vi "LHF.DB.Mongo.Collection.Aggregate.vi"(6 "Extract _id (T)":bool=TRUE, 7 "return type":variant, 8 "error in (no error)":errorcluster, 9 "Operations":variant[](array[variant]), 10 "Collection":string, 11 "LHF.DB.Mongo in":refnum<class "LHF.DB.Mongo.lvclass">) -> (0 "error out":errorcluster, 1 "_id Array":string[](array[string]), 2 "Documents":variant[](array[variant]), 3 "LHF.DB.Mongo out":refnum<class "LHF.DB.Mongo.lvclass">)   [LabVIEW 2013, in "LHF.DB.Mongo.lvclass"]
doc: "return type: wire cluster of expected document output, then variant to data with documents output. use cluster element's name to choose what document field you're expecting\noperations: wire array of cluster variant, name the cluster variant with the desired aggregation operation as $project or $match then use element names to setup pipeline."
uses:
  LHF.DB.Mongo.lvclass
  C:/Users/Ricardo/Desktop/Projetos/LabVIEW-MongoDB/src/Driver/MongoDB.Bson.dll
  Driver/MongoDB.Bson.dll
  <userlib>/_OpenG.lib/string/string.llb/Trim Whitespace (String)__ogtk.vi
  <vilib>/Utility/VariantDataType/VariantType.lvlib
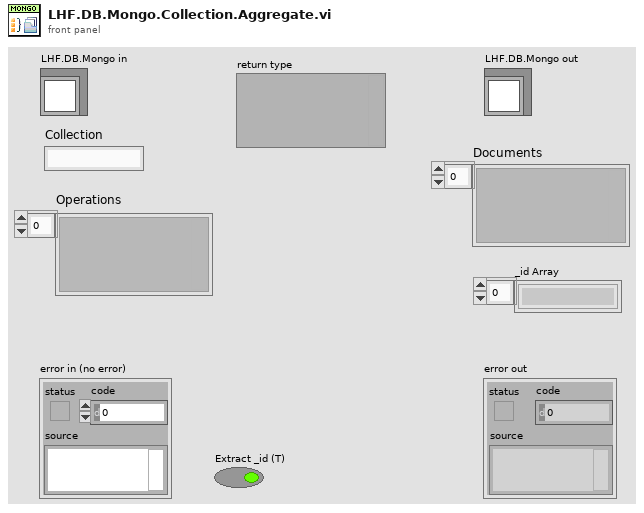
[diagram p1: front panel]
types:
  T1 = enum16{"$project", "$limit", "$skip", "$match", "$redact", "$unwind", "$group", "$sort", "$sample", "$geonear", "$lookup", "$out", "$indexstats"}
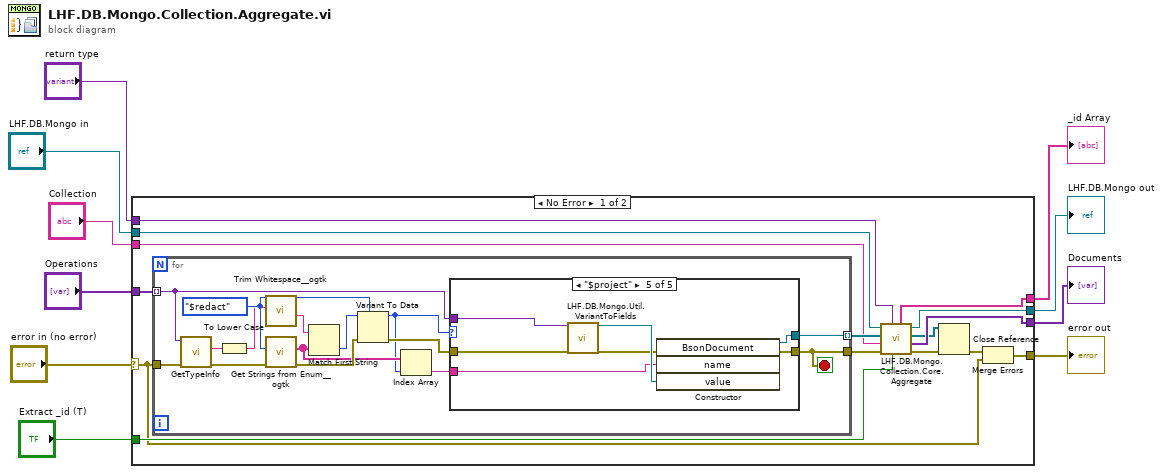
[diagram p0: block diagram]
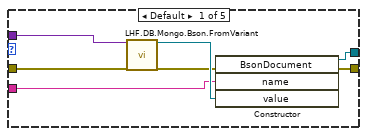
[diagram p2: hidden frame]
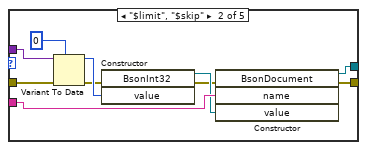
[diagram p3: hidden frame]
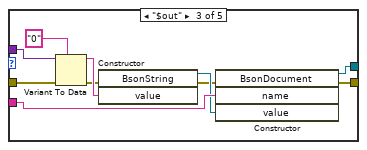
[diagram p4: hidden frame]
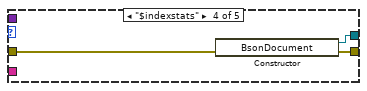
[diagram p5: hidden frame]
diagram:
  n1 = case shown="No Error" "error in (no error)" {
    selector: "error in (no error)" -> [w12 w79]
    tunnel: [w20 w79] -> w9
    tunnel: [w23 w78] -> w7
    tunnel: "LHF.DB.Mongo in" -> [w24 w78]
    tunnel: "Collection" -> [w19 _]
    tunnel: "Operations" -> [w25 _]
    tunnel: [w18 _] -> w4
    tunnel: "Extract _id (T)" -> [w17 _]
    tunnel: [w16 _] -> w2
    tunnel: "return type" -> [w11 _]
    frame No Error {
      n2 = for {
        tunnel: w25 -> [w38] mode=indexing
        tunnel: [w40] -> w21 mode=indexing
        tunnel: [w39] -> w22
        tunnel: w12 -> [w31]
        stop <- w39 stop-if-true
        w37 = T1."$redact"
        n3 = call <vilib>:"GetTypeInfo.vi"("error in (no error)"=w31, "Variant"=w38) -> ("error out"=w32:errorcluster, "Name"=w34:string)  [unwired: 5 in, 3 out]
        n4 = To Lower Case(string=w34) -> (all lower case string=w26:string)
        n5 = call-poly <userlib>:"Trim Whitespace__ogtk.vi"("String in"=w26) -> ("String out"=w35:string)  [unwired: 6 in]
        n6 = call <userlib>:"Get Strings from Enum__ogtk.vi"("error in (no error)"=w32, "Enum"=w37) -> ("error out"=w33:errorcluster, "Enum Strings"=w29:string[])  [unwired: 6 in, 2 out]
        n7 = Match First String(2:w29, 3:w35) -> (0:w36:i32)  [unwired: 1 out]
        n8 = Variant To Data(error in=w33, type=w37, Variant=w36) -> (data=w28:T1, error out=w30:errorcluster)
        n9 = Index Array(array=w29, index=w28) -> (element=w27:string)
        n10 = case shown="\"$project\"" w28 {
          tunnel: [w43 w53 w63 w70 w73] -> w40
          tunnel: [w42 w48 w58 w69 w72] -> w39
          tunnel: w30 -> [w46 w55 w65 w68 w77]
          tunnel: w38 -> [w47 w57 w67 _ w76]
          tunnel: w27 -> [w41 w54 w64 _ w71]
          frame Default {
            n11 = call "LHF.DB.Mongo.Bson.FromVariant.vi"("Variant"=w47, "error IO"=w46) -> ("BsonValue"=w45:refnum<k24>, "error IO 2"=w44:errorcluster)  [unwired: 16 in]
            n12 = constructor class="BsonDocument"(error in=w44, "name"=w41, "value"=w45) -> (reference out=w43:refnum<k24>, error out=w42:errorcluster)  [unwired: 2 in, 3 out]
          }
          frame "$limit", "$skip" {
            n13 = Variant To Data(error in=w55, type=0, Variant=w57) -> (data=w52:i32, error out=w51:errorcluster)
            n14 = constructor class="BsonInt32"(error in=w51, "value"=w52) -> (reference out=w50:refnum<k24>, error out=w49:errorcluster)  [unwired: 2 in, 2 out]
            n15 = constructor class="BsonDocument"(error in=w49, "name"=w54, "value"=w50) -> (reference out=w53:refnum<k24>, error out=w48:errorcluster)  [unwired: 2 in, 3 out]
          }
          frame "$out" {
            n16 = Variant To Data(error in=w65, type="0", Variant=w67) -> (data=w62:string, error out=w61:errorcluster)
            n17 = constructor class="BsonString"(error in=w61, "value"=w62) -> (reference out=w60:refnum<k24>, error out=w59:errorcluster)  [unwired: 2 in, 2 out]
            n18 = constructor class="BsonDocument"(error in=w59, "name"=w64, "value"=w60) -> (reference out=w63:refnum<k24>, error out=w58:errorcluster)  [unwired: 2 in, 3 out]
          }
          frame "$indexstats" {
            n19 = constructor class="BsonDocument"(error in=w68) -> (reference out=w70:refnum<k24>, error out=w69:errorcluster)  [unwired: 2 in, 1 out]
          }
          frame "$project" {
            n20 = call "LHF.DB.Mongo.Util.VariantToFields.vi"("projection type"=w76, "error in (no error)"=w77) -> ("BsonDocument"=w75:refnum<k24>, "error out"=w74:errorcluster)  [unwired: 16 in]
            n21 = constructor class="BsonDocument"(error in=w74, "name"=w71, "value"=w75) -> (reference out=w73:refnum<k24>, error out=w72:errorcluster)  [unwired: 2 in, 3 out]
          }
        }
      }
      n22 = call "LHF.DB.Mongo.Collection.Core.Aggregate.vi"("Extract _id"=w17, "type"=w11, "error in (no error)"=w22, "Collection"=w19, "operations"=w21, "LHF.DB.Mongo in"=w24) -> ("error out"=w14:errorcluster, "Documents"=w18:variant[], "operations out"=w15:refnum<k24>[], "LHF.DB.Mongo out"=w23:refnum<class "LHF.DB.Mongo.lvclass">, "_id Array"=w16:string[])  [unwired: 1 in]
      n23 = Close Reference(reference=w15, error in (no error)=w14) -> (error out=w13:errorcluster)
      n24 = Merge Errors(w13, w12) -> (w20:errorcluster)
    }
    frame Error {
    }
  }
  "error out" <- w9
  "LHF.DB.Mongo out" <- w7
  "Documents" <- w4
  "_id Array" <- w2
